vi "Create Manual Report.vi"() -> ()   [LabVIEW 2013]
doc: "This example illustrates how to create a JUnit test report for a manually defined test suite."
uses:
  <vilib>/addons/_JKI Toolkits/Caraya/classes/Test Suite/Test Suite.lvclass
  JUnit for Azure Pipelines/JUnit for Azure Pipelines.lvclass
  <vilib>/addons/_JKI Toolkits/Caraya/classes/Test Suite/Define Test Suite (Default).vi
  <vilib>/addons/_JKI Toolkits/Caraya/classes/Assert/Assert True.vi
  <vilib>/addons/_JKI Toolkits/Caraya/classes/Test Report/Test Report.lvclass
  <vilib>/addons/_JKI Toolkits/Caraya/classes/Test/Test.lvclass
  <vilib>/addons/_JKI Toolkits/Caraya/classes/Assert/Assert.lvclass
panel:
  out "error out":errorcluster
  in  "Path":path
  # "1) Specify a path to store the test report file.\n2) Run the VI and review the created file.\n\nSee the block diagram for more information."
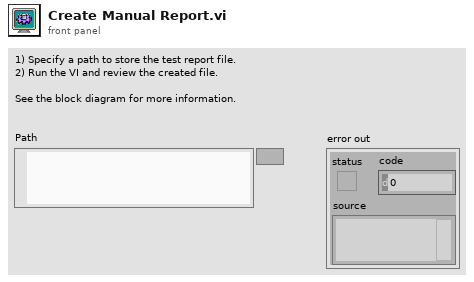
[diagram p1: front panel]
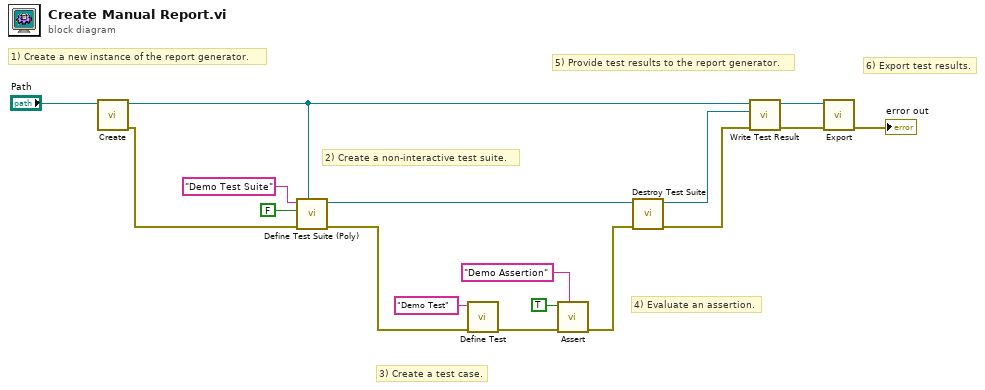
[diagram p0: block diagram]
diagram:
  # "6) Export test results."
  # "5) Provide test results to the report generator."
  # "4) Evaluate an assertion."
  # "3) Create a test case."
  # "2) Create a non-interactive test suite."
  # "1) Create a new instance of the report generator."
  n1 = call "Create.vi"("Path"="Path") -> ("error out"=w3:errorcluster, "JUnit for Azure Pipelines"=w2:refnum<class "JUnit for Azure Pipelines.lvclass">)  [unwired: 9 in]
  n2 = call-poly <vilib>:"Define Test Suite (Poly).vi"("Test Report (optional)"=w2, "error in (no error)"=w3, "Interactive"=FALSE, "Label (VI Title)"="Demo Test Suite") -> ("error out"=w8:errorcluster, "Test Suite"=w14:refnum<class "Test Suite.lvclass">)  [unwired: 5 in, 1 out]
  n3 = call <vilib>:"Define Test.vi"("error in (no error)"=w8, "Label (VI Title)"="Demo Test") -> ("error out"=w9:errorcluster)  [unwired: 8 in, 1 out]
  n4 = call-poly <vilib>:"Assert.vi"("Label"="Demo Assertion" ("Label (VI Title)"), "error in (no error)"=w9, "True?"=TRUE) -> ("error out"=w7:errorcluster)  [unwired: 7 in, 1 out]
  n5 = call-dynamic "Destroy Test Suite.vi"("error in (no error)"=w7, "Test Suite in"=w14) -> ("error out"=w5:errorcluster, "Test Suite Results"=w12:refnum<class "Test Result.lvclass">)  [unwired: 8 in]
  n6 = call <vilib>:"Write Test Result.vi"("error in (no error)"=w5, "Test Result"=w12, "Test Report in"=w2) -> ("error out"=w4:errorcluster, "Test Report out"=w13:refnum<class "JUnit for Azure Pipelines.lvclass">)  [unwired: 7 in]
  n7 = call-dynamic "Export.vi"("error in (no error)"=w4, "JUnit for Azure Pipelines in"=w13) -> ("error out"=→"error out":errorcluster)  [unwired: 8 in, 1 out]
